vi "Drive Encoders.vi"(8 "Reset Encoders?":bool, 9 "Digital Module A":T2={"DIO Module"=enum."Digital Module 2", "Left Encoder B Channel"=enum."DIO 1", "Left Encoder A Channel"=enum."DIO 2", "Right Encoder B Channel"=enum."DIO 3", "Right Encoder A Channel"=enum."DIO 4", "Arm Encoder A Channel"=enum."DIO 5", "Arm Encoder B Channel"=enum."DIO 6", "Pressure Switch"=enum."DIO 7", "Unassigned"=enum."DIO 8", "Unassigned"=enum."DIO 9", "Ultrasonic Trigger"=enum."DIO 10", "Remus Switch"=enum."DIO 11", "Unassigned"=enum."DIO 12", "Unassigned"=enum."DIO 13", "Unassigned"=enum."DIO 14"}, 10 "Remus?":bool, 11 "Mode":enum16{"Init", "Run", "End"}(ring)) -> (0 "Right-Left":dbl, 1 "Average Distance":dbl, 2 "Average FPS":dbl, 3 "Distance":T1, 4 "Rate FeetPerSec":cluster{"Left Rate":dbl, "Right Rate":dbl}, 6 "Rate InchPerSec":cluster{"Left Rate":dbl, "Right Rate":dbl})   [LabVIEW 2013]
doc: "Setup and get the Drive Encoders"
uses:
  <vilib>/Rock Robotics/WPI/Encoder/WPI_EncoderType.ctl
  Type Defs/Digital Module A.ctl
  <vilib>/Rock Robotics/SystemInterfaces/Typedef/FPGA_TypedefDigitalModule.ctl
  <vilib>/Rock Robotics/SystemInterfaces/DIO/FPGA_DIOChannel.ctl
  <vilib>/Rock Robotics/WPI/Counter/WPI_CounterDigitalInputToDigitalSource.vi
panel:
  in  "Encoder CPR":dbl=250.0
  in  "Wheel diameter (in)":dbl=6.0
  in  "Number Samples to Average":u8=1 min=1 max=128
  in  "Decoding Type":T5=enum."4x"
  in  "Minimum Rate":dbl=20.0
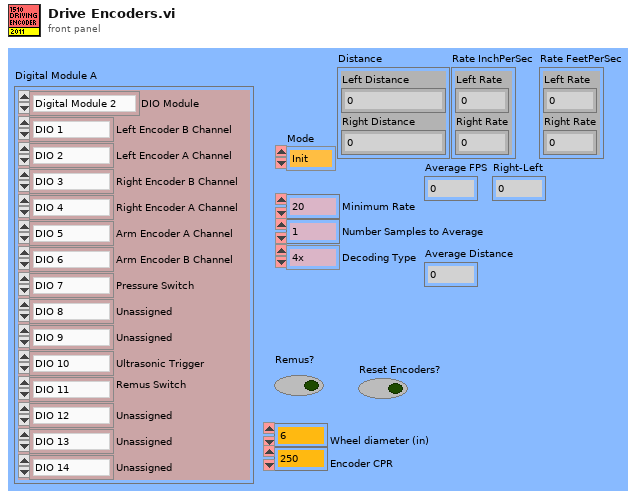
[diagram p1: front panel]
types:
  T1 = cluster{"Left Distance":dbl, "Right Distance":dbl}
  T2 = typedef "Digital Module A.ctl" = cluster{"DIO Module":T3, "Left Encoder B Channel":T4, "Left Encoder A Channel":T4, "Right Encoder B Channel":T4, "Right Encoder A Channel":T4, "Arm Encoder A Channel":T4, "Arm Encoder B Channel":T4, "Pressure Switch":T4, "Unassigned":T4, "Unassigned":T4, "Ultrasonic Trigger":T4, "Remus Switch":T4, "Unassigned":T4, "Unassigned":T4, "Unassigned":T4}
  T3 = typedef "FPGA_TypedefDigitalModule.ctl" = enum16{"Digital Module 1", "Digital Module 2"}
  T4 = typedef "FPGA_DIOChannel.ctl" = enum8{"DIO 1", "DIO 2", "DIO 3", "DIO 4", "DIO 5", "DIO 6", "DIO 7", "DIO 8", "DIO 9", "DIO 10", "DIO 11", "DIO 12", "DIO 13", "DIO 14", "Invalid"}
  T5 = typedef "WPI_EncoderType.ctl" = enum16{"1x", "2x", "4x"}
  T6 = typedef "WPI_DigitalInputDevRef.ctl" = cluster{"DevStatus":errorcluster, "DIO Channel":T4, "Digital Module":T3}
  T7 = typedef "FPGA_CounterEncoderSourceConvertionLVSourceType.ctl" = cluster{"DevStatus":errorcluster, "AnalogTriggerMode?":bool, "DigitalMode":cluster{"Digital Module":T3, "DIO Channel":T8}, "AnalogTriggerMode":cluster{"AnalogTriggerIndex":T9, "OutputType":T10}}
  T8 = typedef "FPGA_DIODigitalSourceChannel.ctl" = enum8{"DIO 1", "DIO 2", "DIO 3", "DIO 4", "DIO 5", "DIO 6", "DIO 7", "DIO 8", "DIO 9", "DIO 10", "DIO 11", "DIO 12", "DIO 13", "DIO 14", "Disabled"}
  T9 = typedef "FPGA_AnalogTriggerIndex.ctl" = enum8{"Trig 0", "Trig 1", "Trig 2", "Trig 3", "Trig 4", "Trig 5", "Trig 6", "Trig 7", "Invalid"}
  T10 = typedef "FPGA_AnalogTriggerOutType.ctl" = enum16{"InWindow", "TriggerState", "Rising", "Falling"}
  T11 = typedef "WPI_EncoderDevRef.ctl" = cluster{"DevStatus":errorcluster, "EncoderIndex":T12, "CounterIndex":T13, "DistancePerCount":dbl, "Decoding Type":T5}
  T12 = typedef "FPGA_EncoderIdx.ctl" = enum8{"Enc 0", "Enc 1", "Enc 2", "Enc 3", "Invalid"}
  T13 = typedef "FPGA_CounterCtrSystemIndex.ctl" = enum8{"Ctr 0", "Ctr 1", "Ctr 2", "Ctr 3", "Ctr 4", "Ctr 5", "Ctr 6", "Ctr 7", "Invalid"}
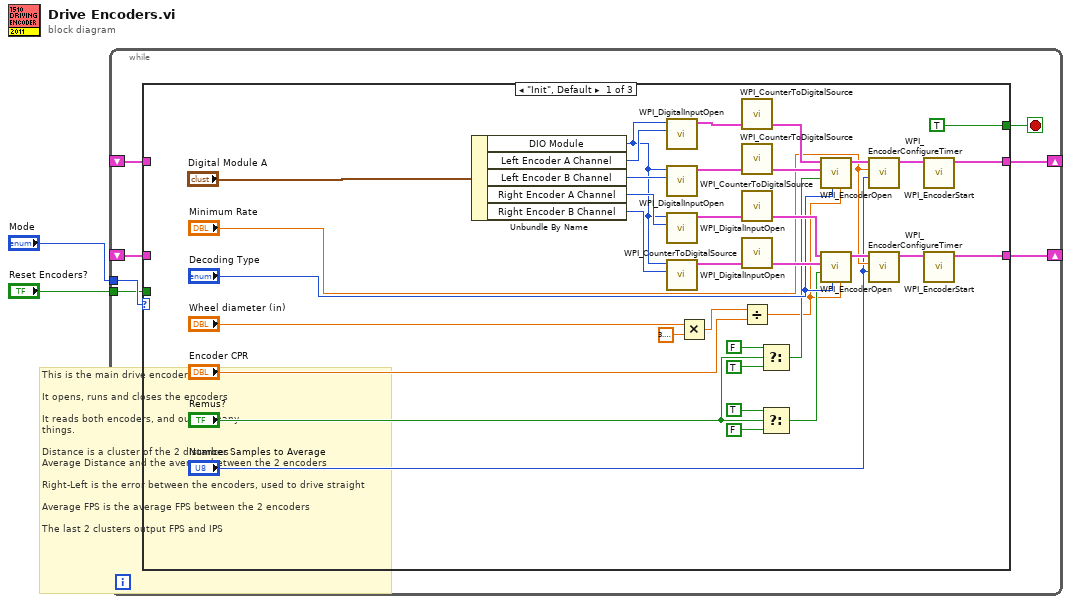
[diagram p0: block diagram]
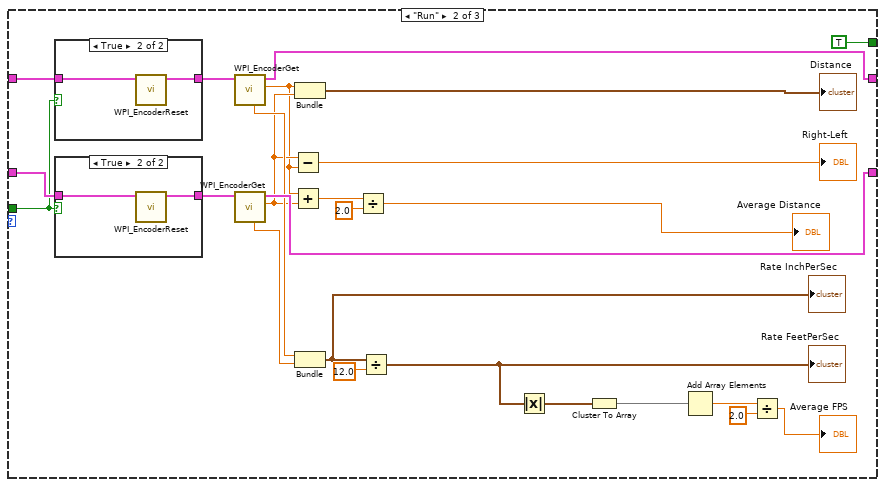
[diagram p2: hidden frame]
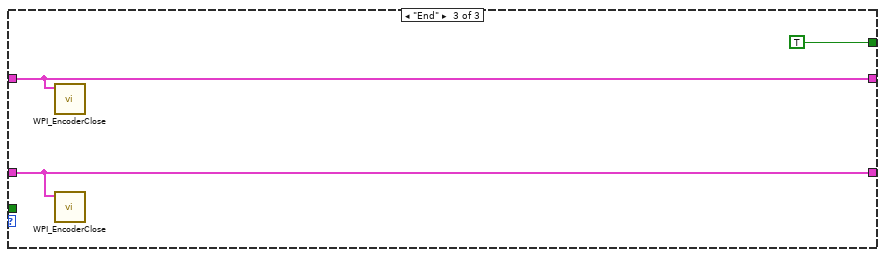
[diagram p5: hidden frame]
diagram:
  # "This is the main drive encoder VI\n\nIt opens, runs and closes the encoders\n\nIt reads both encoders, and output many\nthings.\n\nDistance is a cluster of the 2 distances\nAverage Distance and the average between the 2 encoders\n\nRight-Left is the error between the encoders, used to drive straight\n\nAverage FPS is the average FPS between the 2 encoders\n\nThe last 2 clusters output FPS and IPS"
  n1 = while {
    tunnel: "Mode" -> [w4]
    shift-right: [w8] -> _
    shift-left: _ -> [w6]
    shift-right: [w9] -> _
    shift-left: _ -> [w7]
    tunnel: "Reset Encoders?" -> [w3]
    stop <- w5 stop-if-true
    n2 = case shown="\"Init\", Default" w4 {
      tunnel: [w23 w65 w78] -> w9
      tunnel: [w22 w64 w79] -> w8
      tunnel: w7 -> [_ w70 w78]
      tunnel: w6 -> [_ w69 w79]
      tunnel: [TRUE TRUE TRUE] -> w5
      tunnel: w3 -> [_ w63 _]
      frame "Init", Default {
        n3 = Unbundle By Name("Digital Module A") -> ("DIO Module"=w27:T3, "Left Encoder A Channel"=w32:T4, "Left Encoder B Channel"=w31:T4, "Right Encoder A Channel"=w30:T4, "Right Encoder B Channel"=w28:T4)
        n4 = call <vilib>:"WPI_DigitalInputOpen.vi"("DIO Channel"=w32, "Digital Module (Module 1)"=w27) -> ("DigitalInputDevRef"=w36:T6)  [unwired: 1 in, 8 out]
        n5 = call <vilib>:"WPI_DigitalInputOpen.vi"("DIO Channel"=w31, "Digital Module (Module 1)"=w27) -> ("DigitalInputDevRef"=w35:T6)  [unwired: 1 in, 8 out]
        n6 = call <vilib>:"WPI_DigitalInputOpen.vi"("DIO Channel"=w30, "Digital Module (Module 1)"=w27) -> ("DigitalInputDevRef"=w41:T6)  [unwired: 1 in, 8 out]
        n7 = call <vilib>:"WPI_DigitalInputOpen.vi"("DIO Channel"=w28, "Digital Module (Module 1)"=w27) -> ("DigitalInputDevRef"=w40:T6)  [unwired: 1 in, 8 out]
        n8 = Multiply(x="Wheel diameter (in)", y=3.141592653589793) -> (x*y=w13:dbl)
        n9 = call-poly <vilib>:"WPI_CounterToDigitalSource.vi"("DigitalInputDevRef"=w36) -> ("Digital Source"=w37:T7)  [unwired: 6 out]
        n10 = call-poly <vilib>:"WPI_CounterToDigitalSource.vi"("DigitalInputDevRef"=w35) -> ("Digital Source"=w34:T7)  [unwired: 6 out]
        n11 = call-poly <vilib>:"WPI_CounterToDigitalSource.vi"("DigitalInputDevRef"=w41) -> ("Digital Source"=w42:T7)  [unwired: 1 in, 5 out]
        n12 = call-poly <vilib>:"WPI_CounterToDigitalSource.vi"("DigitalInputDevRef"=w40) -> ("Digital Source"=w43:T7)  [unwired: 6 out]
        n13 = Divide(x=w13, y="Encoder CPR") -> (x/y=w11:dbl)
        n14 = Select(t=FALSE, s="Remus?", f=TRUE) -> (s? t:f=w21:bool)
        n15 = Select(t=TRUE, s="Remus?", f=FALSE) -> (s? t:f=w18:bool)
        n16 = call <vilib>:"WPI_EncoderOpen.vi"("DistancePerCount"=w11, "Decoding Type"="Decoding Type", "Invert Direction (False)"=w21, "BSource"=w34, "ASource"=w37) -> ("EncoderDevRef"=w39:T11)  [unwired: 3 in, 3 out]
        n17 = call <vilib>:"WPI_EncoderOpen.vi"("DistancePerCount"=w11, "Decoding Type"="Decoding Type", "Invert Direction (False)"=w18, "BSource"=w43, "ASource"=w42) -> ("EncoderDevRef"=w44:T11)  [unwired: 3 in, 3 out]
        n18 = call <vilib>:"WPI_EncoderConfigureTimer.vi"("Number Samples to Average"="Number Samples to Average", "Minimum Rate"="Minimum Rate", "EncoderDevRef"=w39) -> ("EncoderDevRef"=w38:T11)  [unwired: 1 in, 7 out]
        n19 = call <vilib>:"WPI_EncoderConfigureTimer.vi"("Number Samples to Average"="Number Samples to Average", "Minimum Rate"="Minimum Rate", "EncoderDevRef"=w44) -> ("EncoderDevRef"=w45:T11)  [unwired: 1 in, 7 out]
        n20 = call <vilib>:"WPI_EncoderStart.vi"("EncoderDevRef"=w38) -> ("EncoderDevRef"=w23:T11)  [unwired: 1 in, 9 out]
        n21 = call <vilib>:"WPI_EncoderStart.vi"("EncoderDevRef"=w45) -> ("EncoderDevRef"=w22:T11)  [unwired: 1 in, 9 out]
      }
      frame "Run" {
        n22 = case shown="True" w63 {
          tunnel: w70 -> [w74 w76]
          tunnel: [w74 w75] -> w67
          frame False {
          }
          frame True {
            n23 = call <vilib>:"WPI_EncoderReset.vi"("EncoderDevRef"=w76) -> ("EncoderDevRef"=w75:T11)  [unwired: 1 in, 9 out]
          }
        }
        n24 = case shown="True" w63 {
          tunnel: w69 -> [w71 w73]
          tunnel: [w71 w72] -> w66
          frame False {
          }
          frame True {
            n25 = call <vilib>:"WPI_EncoderReset.vi"("EncoderDevRef"=w73) -> ("EncoderDevRef"=w72:T11)  [unwired: 1 in, 9 out]
          }
        }
        n26 = call <vilib>:"WPI_EncoderGet.vi"("EncoderDevRef"=w67) -> ("Distance"=w47:dbl, "EncoderDevRef"=w65:T11, "Rate"=w61:dbl)  [unwired: 1 in, 7 out]
        n27 = call <vilib>:"WPI_EncoderGet.vi"("EncoderDevRef"=w66) -> ("Distance"=w48:dbl, "EncoderDevRef"=w64:T11, "Rate"=w60:dbl)  [unwired: 1 in, 7 out]
        n28 = Subtract(x=w48, y=w47) -> (x-y=→"Right-Left":dbl)
        n29 = Add(x=w47, y=w48) -> (x+y=w51:dbl)
        n30 = Bundle("Distance"=w47, "Distance"=w48) -> (→"Distance":cluster{"Distance":dbl, "Distance":dbl})  [unwired: 1 out]
        n31 = Bundle("Rate"=w61, "Rate"=w60) -> (w59:cluster{"Rate":dbl, "Rate":dbl})  [unwired: 1 out]
        "Rate InchPerSec" <- w59
        n32 = Divide(x=w51, y=2.0) -> (x/y=→"Average Distance":dbl)
        n33 = Divide(x=w59, y=12.0) -> (x/y=w57:cluster{"Rate":dbl, "Rate":dbl})
        "Rate FeetPerSec" <- w57
        n34 = Absolute Value(x=w57) -> (abs(x)=w56:cluster{"Rate":dbl, "Rate":dbl})
        n35 = Cluster To Array(cluster=w56) -> (array=w55:dbl[])
        n36 = Add Array Elements(numeric array=w55) -> (sum=w54:dbl)
        n37 = Divide(x=w54, y=2.0) -> (x/y=→"Average FPS":dbl)
      }
      frame "End" {
        n38 = call <vilib>:"WPI_EncoderClose.vi"("EncoderDevRef"=w78) -> ()  [unwired: 2 in, 9 out]
        n39 = call <vilib>:"WPI_EncoderClose.vi"("EncoderDevRef"=w79) -> ()  [unwired: 2 in, 9 out]
      }
    }
  }
